vi "_Get or Add Row.vi"(8 "error in":errorcluster, 10 "Row Index":i32, 11 "Worksheetpart in":refnum<k24>) -> (0 "error out":errorcluster, 2 "Row":refnum<k24>, 3 "WorksheetPart out":refnum<k24>)   [LabVIEW 2021, in "Open Xml.lvlib"]
uses:
  Open Xml.lvlib
  D:/git/Open-Xml-LabVIEW/dll/DocumentFormat.OpenXml.dll
  dll/DocumentFormat.OpenXml.dll
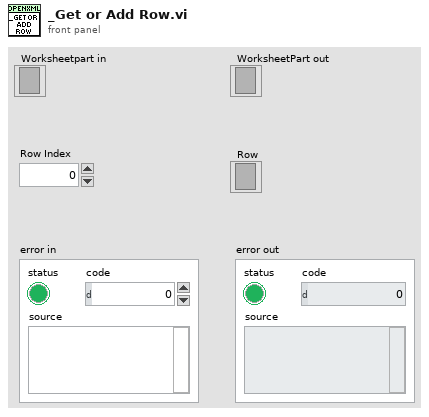
[diagram p1: front panel]
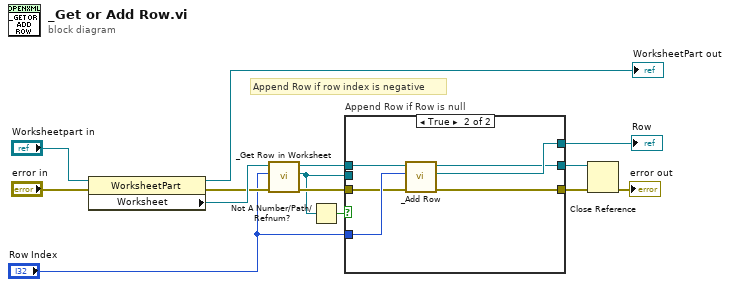
[diagram p0: block diagram]
diagram:
  # "Append Row if row index is negative"
  n1 = property class="WorksheetPart"(reference="Worksheetpart in", error in="error in") -> (reference out=→"WorksheetPart out":refnum<k24>, error out=w9:errorcluster, "Worksheet"=w10:refnum<k24>)
  n2 = call "_Get Row in Worksheet.vi"("error in"=w9, "RowIndex"="Row Index", "Worksheet in"=w10) -> ("error out"=w7:errorcluster, "Row out"=w3:refnum<k24>, "Worksheet out"=w6:refnum<k24>)  [unwired: 6 in]
  n3 = Not A Number/Path/Refnum?(number/path/refnum=w3) -> (NaN/Path/Refnum?=w11:bool)
  n4 = case "Append Row if Row is null" shown="True" w11 {
    tunnel: "Row Index" -> [_ w23]
    tunnel: w7 -> [w17 w22]
    tunnel: w6 -> [w15 w21]
    tunnel: [w17 w20] -> w5
    tunnel: [w16 w19] -> w4
    tunnel: w3 -> [w16 _]
    tunnel: [w15 w18] -> w1
    frame False {
    }
    frame True {
      n5 = call "_Add Row.vi"("error in"=w22, "RowIndex"=w23, "Worksheet in"=w21) -> ("error out"=w20:errorcluster, "Row"=w19:refnum<k24>, "Worksheet out"=w18:refnum<k24>)  [unwired: 6 in]
    }
  }
  "Row" <- w4
  n6 = Close Reference(reference=w1, error in (no error)=w5) -> (error out=→"error out":errorcluster)
